vi "Instrument Read-Write.vi"(0 "VISA resource In":refnum<visa-resource-name>, 5 "String To Write":string, 11 "error in (no error)":errorcluster) -> (4 "VISA resource Out":refnum<visa-resource-name>, 6 "Data Read":string, 15 "error out":errorcluster)   [LabVIEW 2018]
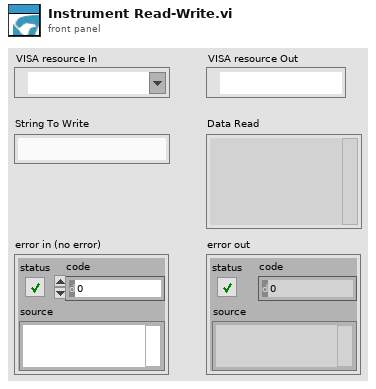
[diagram p1: front panel]
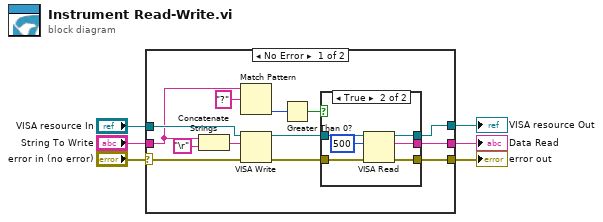
[diagram p0: block diagram]
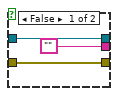
[diagram p2: hidden frame]
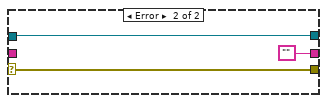
[diagram p3: hidden frame]
diagram:
  n1 = case shown="No Error" "error in (no error)" {
    selector: "error in (no error)" -> [w19 w31]
    tunnel: [w13 w31] -> w5
    tunnel: "String To Write" -> [w7 _]
    tunnel: "VISA resource In" -> [w18 w30]
    tunnel: [w11 w30] -> w2
    tunnel: [w10 ""] -> w1
    frame No Error {
      n2 = Concatenate Strings(w7, "\r") -> (w9:string)
      n3 = Match Pattern(string=w7, regular expression="?") -> (offset past match=w16:i32)  [unwired: 1 in, 3 out]
      n4 = VISA Write(VISA resource name=w18, write buffer=w9, error in (no error)=w19) -> (VISA resource name out=w12:refnum<visa-resource-name>, error out=w14:errorcluster)  [unwired: 1 out]
      n5 = Greater Than 0?(x=w16) -> (x > 0?=w15:bool)
      n6 = case shown="True" w15 {
        tunnel: w14 -> [w22 w28]
        tunnel: [w22 w27] -> w13
        tunnel: w12 -> [w21 w26]
        tunnel: [w21 w25] -> w11
        tunnel: ["" w24] -> w10
        frame False {
        }
        frame True {
          n7 = VISA Read(VISA resource name=w26, byte count=u32 500, error in (no error)=w28) -> (VISA resource name out=w25:refnum<visa-resource-name>, read buffer=w24:string, error out=w27:errorcluster)  [unwired: 1 out]
        }
      }
    }
    frame Error {
    }
  }
  "error out" <- w5
  "Data Read" <- w1
  "VISA resource Out" <- w2
